vi "SetupTiming.vi"(8 "error in (no error)":errorcluster, 11 "ClassIn":refnum<class "NiPxi6733.lvclass">) -> (0 "error out":errorcluster, 3 "ClassOut":refnum<class "NiPxi6733.lvclass">)   [LabVIEW 2014, in "FGenPlugins.lvlib" / "NiPxi6733.lvclass"]
uses:
  NiPxi6733.lvclass
  NiPxi6733.lvclass/NiPxi6733.ctl
  Accessors/Read Timebase.vi
  <vilib>/DAQmx/configure/timing.llb/DAQmx Timing (Sample Clock).vi
  <resource>/objmgr/daqmx.rc
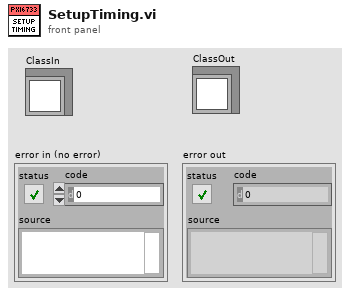
[diagram p1: front panel]
types:
  T1 = typedef "FGenPlugins.lvlib/NISTFGenPluginsBase.lvclass/ChannelParamElement.ctl" = cluster{"sName":string, "eOperateMode":u16, "bEnabled":bool, "eOutputMode":u16, "iIndex":i32, "iNameBufferSize":i32, "fGain":dbl}
  T2 = typedef "FGenPlugins.lvlib/NISTFGenPluginsBase.lvclass/StdWaveformParams.ctl" = cluster{"eWaveform":u16, "dAmplitude":dbl, "dDcOffset":dbl, "dFrequency":dbl, "dStartPhase":dbl, "dSampleRate":dbl, "dNumSamples":dbl}
  T3 = typedef "FGenPlugins.lvlib/NISTFGenPluginsBase.lvclass/ArbWfrmParams.ctl" = cluster{"sWfrmHandle":string, "iSize":i32, "dData":dbl[], "dGain":dbl, "dOffset":dbl, "dSampleRate":dbl}
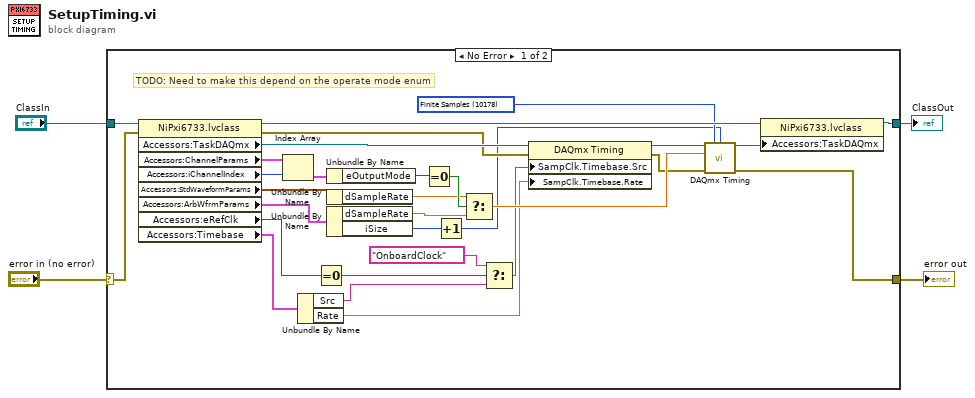
[diagram p0: block diagram]
diagram:
  n1 = case shown="No Error" "error in (no error)" {
    selector: "error in (no error)" -> [w33 w36]
    tunnel: "ClassIn" -> [w34 w35]
    tunnel: [w18 w36] -> w2
    tunnel: [w17 w35] -> w1
    frame No Error {
      w16 = 10178 items=["Finite Samples"=10178, "Continuous Samples"=10123, "Hardware Timed Single Point"=12522] ("sample mode")
      # "TODO: Need to make this depend on the operate mode enum"
      n2 = property class="NiPxi6733.lvclass"(reference=w34, error in=w33) -> (reference out=w20:refnum<class "NiPxi6733.lvclass">, error out=w7:errorcluster, "Accessors:TaskDAQmx"=w23:refnum<k21>, "Accessors:ChannelParams"=w32:T1[], "Accessors:iChannelIndex"=w31:i32, "Accessors:StdWaveformParams"=w29:T2, "Accessors:ArbWfrmParams"=w28:T3, "Accessors:eRefClk"=w8:u16, "Accessors:Timebase"=w11:cluster{"Src":tag, "Rate":dbl})
      n3 = Index Array(array=w32, index=w31) -> (element=w30:T1)
      n4 = Unbundle By Name(w11) -> ("Src"=w9:tag, "Rate"=w10:dbl)
      n5 = Equal To 0?(x=w8) -> (x = 0?=w14:bool)
      n6 = Unbundle By Name(w30) -> ("eOutputMode"=w27:u16)
      n7 = Unbundle By Name(w29) -> ("dSampleRate"=w25:dbl)
      n8 = Unbundle By Name(w28) -> ("dSampleRate"=w24:dbl, "iSize"=w12:i32)
      n9 = Equal To 0?(x=w27) -> (x = 0?=w26:bool)
      n10 = Increment(x=w12) -> (x+1=w5:i32)
      n11 = Select(t=w25, s=w26, f=w24) -> (s? t:f=w22:dbl)
      n12 = Select(t=tag "OnboardClock" ("source"), s=w14, f=w9) -> (s? t:f=w13:tag)
      n13 = property class="DAQmx Timing"(reference=w23, error in=w7, "SampClk.Timebase.Src"=w13, "SampClk.Timebase.Rate"=w10) -> (reference out=w15:refnum<k21>, error out=w6:errorcluster)
      n14 = call-poly <vilib>:"DAQmx Timing.vi"("task/channels in"=w15, "sample mode"=w16, "samples per channel"=w5, "rate"=w22, "error in"=w6) -> ("task out"=w19:refnum<k21>, "error out"=w18:errorcluster)  [unwired: 9 in]
      n15 = property class="NiPxi6733.lvclass"(reference=w20, "Accessors:TaskDAQmx"=w19) -> (reference out=w17:refnum<class "NiPxi6733.lvclass">)  [unwired: 1 in, 1 out]
    }
    frame Error {
    }
  }
  "ClassOut" <- w1
  "error out" <- w2
